vi "PathDrawerMain.vi"() -> ()   [LabVIEW 2017]
uses:
  Dawgma Programming Library/Controls/PurePursuit/PathFileData.ctl
  Dawgma Programming Library/Controls/PurePursuit/RobotNeededPathData.ctl
panel:
  in  "Tab Control":enum32{"Path", "Load/Save"}(tab)
  in  "Deaccel":dbl=50.0 format="%#_13g"
  in  "SlowSpeed":dbl=15.0 format="%#_13g"
  in  "SlowDistanceAtEnd":dbl=12.0 format="%#_13g"
  in  "Speed/Curve":dbl=2.0 format="%#_13g"
  in  "DriveBackwards?":bool
  in  "Lookahead":dbl=13.0
  out "Points (in)":cluster{dbl, dbl}[](array[cluster])=[{14.875179340028694, 248.22955523672883}, {20.874656142200276, 248.30358846723587}, {26.874111844136586, 248.37762105138137}, {32.87350807743945, 248.45164576572313}, {38.87285031681461, 248.52564930010115}, {44.8721376174185, 248.59961966708173}, {50.87132679490307, 248.67354461649725}, {56.87033754344792, 248.74740402354425}, {62.86906734714655, 248.82116341910367}, {68.86738582507886, 248.8947700228471}, {74.8651048928512, 248.9681473786283}, {80.86193607975939, 249.04118420575625}, {86.85743425686633, 249.11371611190245}, {92.85096070503305, 249.18549244057994}, {98.84145913304778, 249.25615421906943}, {104.8276556156584, 249.32512066220386}, {110.80708687815371, 249.39160976611277}, {116.77680979233328, 249.4543515328238}, {122.73186791730424, 249.5115256430506}, {128.6649834222615, 249.56041338385793}, {134.56548779738634, 249.5969246365727}, {140.417375186257, 249.6149706245841}, {146.1966910294908, 249.60548863042237}, {151.86775390690585, 249.55495714900198}, {157.37740484291632, 249.4431992192172}, {162.64635606562646, 249.2401236836006}, {167.55632241578652, 248.9008602167623}, {172.80142342709613, 248.36924030479463}, {178.27099698643164, 247.70868036210402}, {183.89073844553332, 246.9617176111296}, {189.61066276690974, 246.15689887726526}, {195.3970009046773, 245.3134049055755}, {201.22672879119182, 244.44415649854506}, {207.08384341112958, 243.55790546653972}, {212.9567773862825, 242.6606503511154}, {218.83652869344567, 241.75660718632653}, {224.71520193237015, 240.84889249476205}, {230.58472714757215, 239.94002850052652}, {236.43555125878544, 239.03235181687802}, {242.25509137335504, 238.1283916506969}, {248.0256984324822, 237.231278977795}, {253.72180303927817, 236.34525315742894}, {259.30577066584806, 235.47634844945551}, {264.7218219756948, 234.63337048251796}, {269.8869762914892, 233.8293235417345}, {274.67764890352106, 233.08351364924852}, {278.909612625538, 232.42467718794836}]
  in  "Points":cluster{dbl, dbl}[](array[cluster])=[{40.0, 78.0}, {202.0, 76.0}, {324.0, 95.0}]
  in  "Roundedness":dbl(slide)=0.8606565656565657 scale=0.6..0.997
  in  "Length":dbl=38.5
  in  "Width":dbl=33.0
  in  "CenterRotOffset":dbl=15.5
  in  "PointSpacing":dbl=6.0 min=1.0 format="%#_13g"
  in  "Flip Path":bool
  in  "MaxVel":dbl=110.0 format="%#_13g"
  in  "Accel":dbl=50.0 format="%#_13g"
  in  "StartingPosition":enum16{"1", "2", "3", "4", "No Preset"}(ring)
  in  "ExportAllToRobot":bool
  in  "LocalTempPaths":i32(listbox)
  out "standard output":string
  in  "SaveToLocal":bool
  in  "LoadFromLocal":bool
  in  "ExportToRobot":bool
  in  "LoadAllFromRobot":bool
  in  "LocalPaths":i32(listbox)=2
  out "standard error":string="NI Linux Real-Time (run mode)\n\nLog in with your NI-Auth credentials.\n\n"
  in  "LocalFileNames":string[](array[string])=["1A.txt", "1B.txt", "1C.txt", "1D.txt", "2A.txt", "2B.txt", "2C.txt", "2D.txt", "3A.txt", "3B.txt", "3C.txt", "3D.txt", "4A.txt", "4B.txt", "4C.txt", "4D.txt"]
  in  "Stop":bool
  out "Path Drawer":T1(plugin-control)
  # "Includes bumpers"
  # "INSTRUCTIONS"
  # "The red line is the path that the robot recieves. Everything else is to help create that path\n\nUse the multi-line tool to draw a path. Double click to stop drawing.\nHover over a node and press backspace to remove it.\nPress I to insert a new node (at the end of the path only, for now)\n\nUse the contols to input robot width, height, and center of rotation offset,\nHow far apart the points in the \"real world units\" path are,\nWhether the robot travels on the left or right of your green lines, and\nthe roundedness of the path. (Note: point spacing affects roundedness)\n\nYou can manually edit the green node's location in the path with the Points array,\nor drag the nodes on the image\n\nPress Export To File and enter the file name (no extension) to save the path to a file in the\nThisVIsDirectory\\Paths\\ folder\n\nIf you acidentally clear your path press Z quickly to get it back"
  # "Responses of CMDs run"
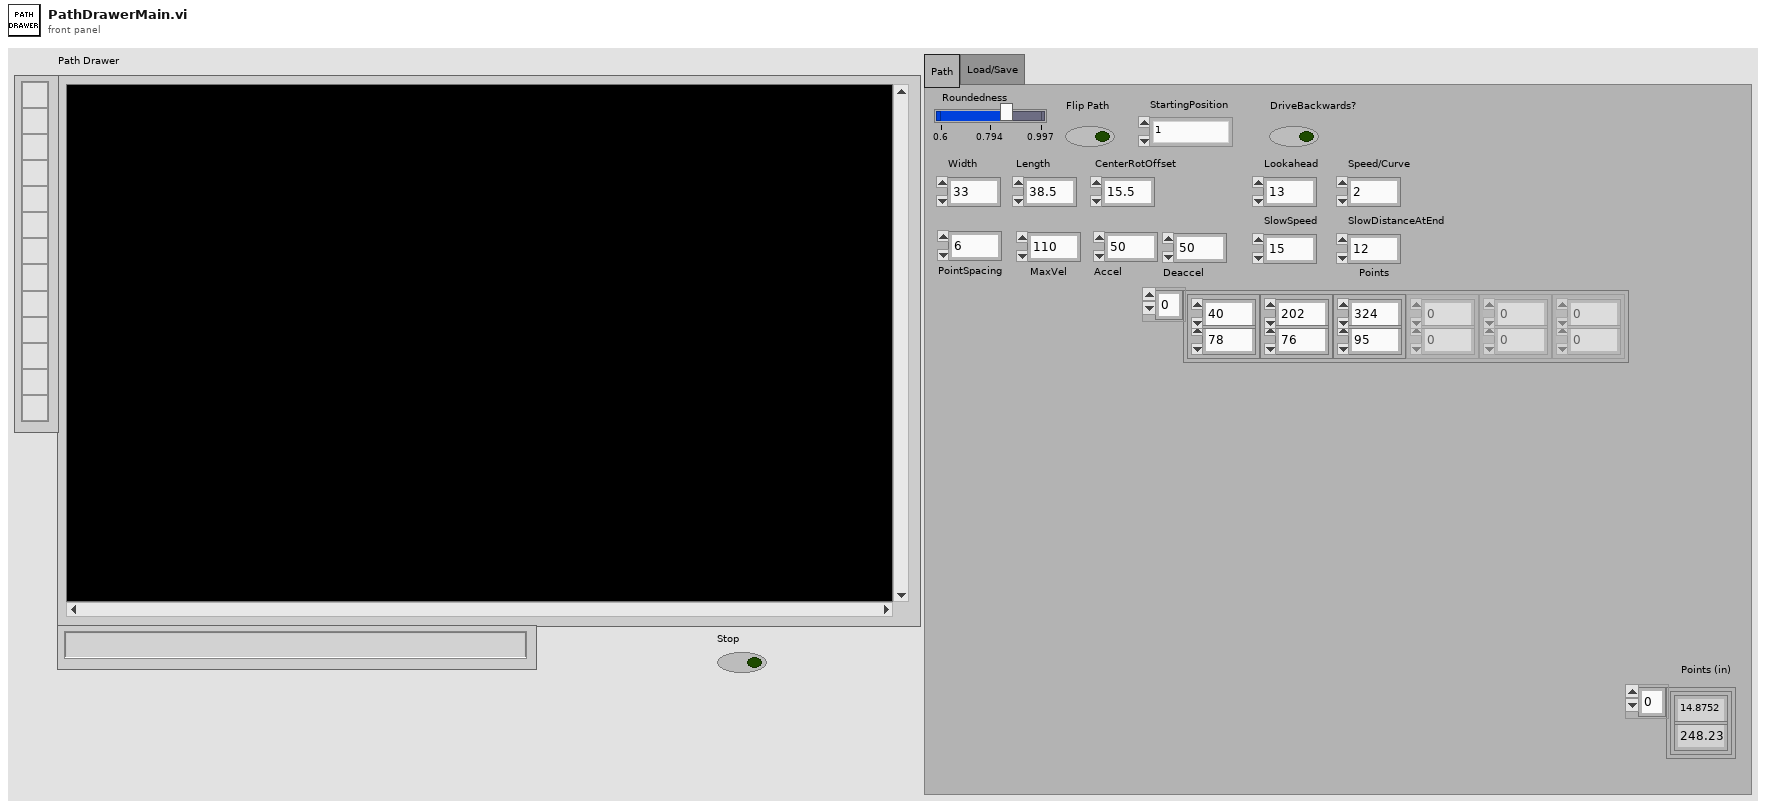
[diagram p1: front panel]
types:
  T1 = typedef "IMAQ Image.ctl" = refnum<image>
  T2 = typedef "Image Type" = u32
  T3 = enum16{"open", "replace", "create", "open or create", "replace or create", "replace or create with confirmation"}
  T4 = cluster{"Global Rectangle":i32[], "Contours":cluster{"Contour Type":u32, "ROI Type":u32, "Points":i32[]}[]}
  T5 = cluster{"Contour Type":u32, "ROI Type":u32, "Points":i32[]}[]
  T6 = cluster{"Contour Type":u32, "ROI Type":u32, "Points":i32[]}
  T7 = typedef "PathFileData.ctl" = cluster{"RobotNeeded":T8, "Meta":cluster{"Path (px)":cluster{i32, i32}[], "RobotWidth":dbl, "RobotLength":dbl, "CenterOfRotYOffset":dbl, "Roundedness":dbl, "StartingPositionPreset":u32, "PathName":string}}
  T8 = typedef "RobotNeededPathData.ctl" = cluster{"Path":cluster{dbl, dbl}[], "MaxVel":dbl, "MaxAccel":dbl, "Backwards?":bool, "PointSpacing":dbl, "LookaheadDist":dbl, "Speed/Curve":dbl, "SlowDistanceAtEnd":dbl, "SlowSpeed":dbl, "MaxDeAccel":dbl}
  T9 = cluster{"Path (px)":cluster{i32, i32}[], "RobotWidth":dbl, "RobotLength":dbl, "CenterOfRotYOffset":dbl, "Roundedness":dbl, "StartingPositionPreset":u32, "PathName":string}
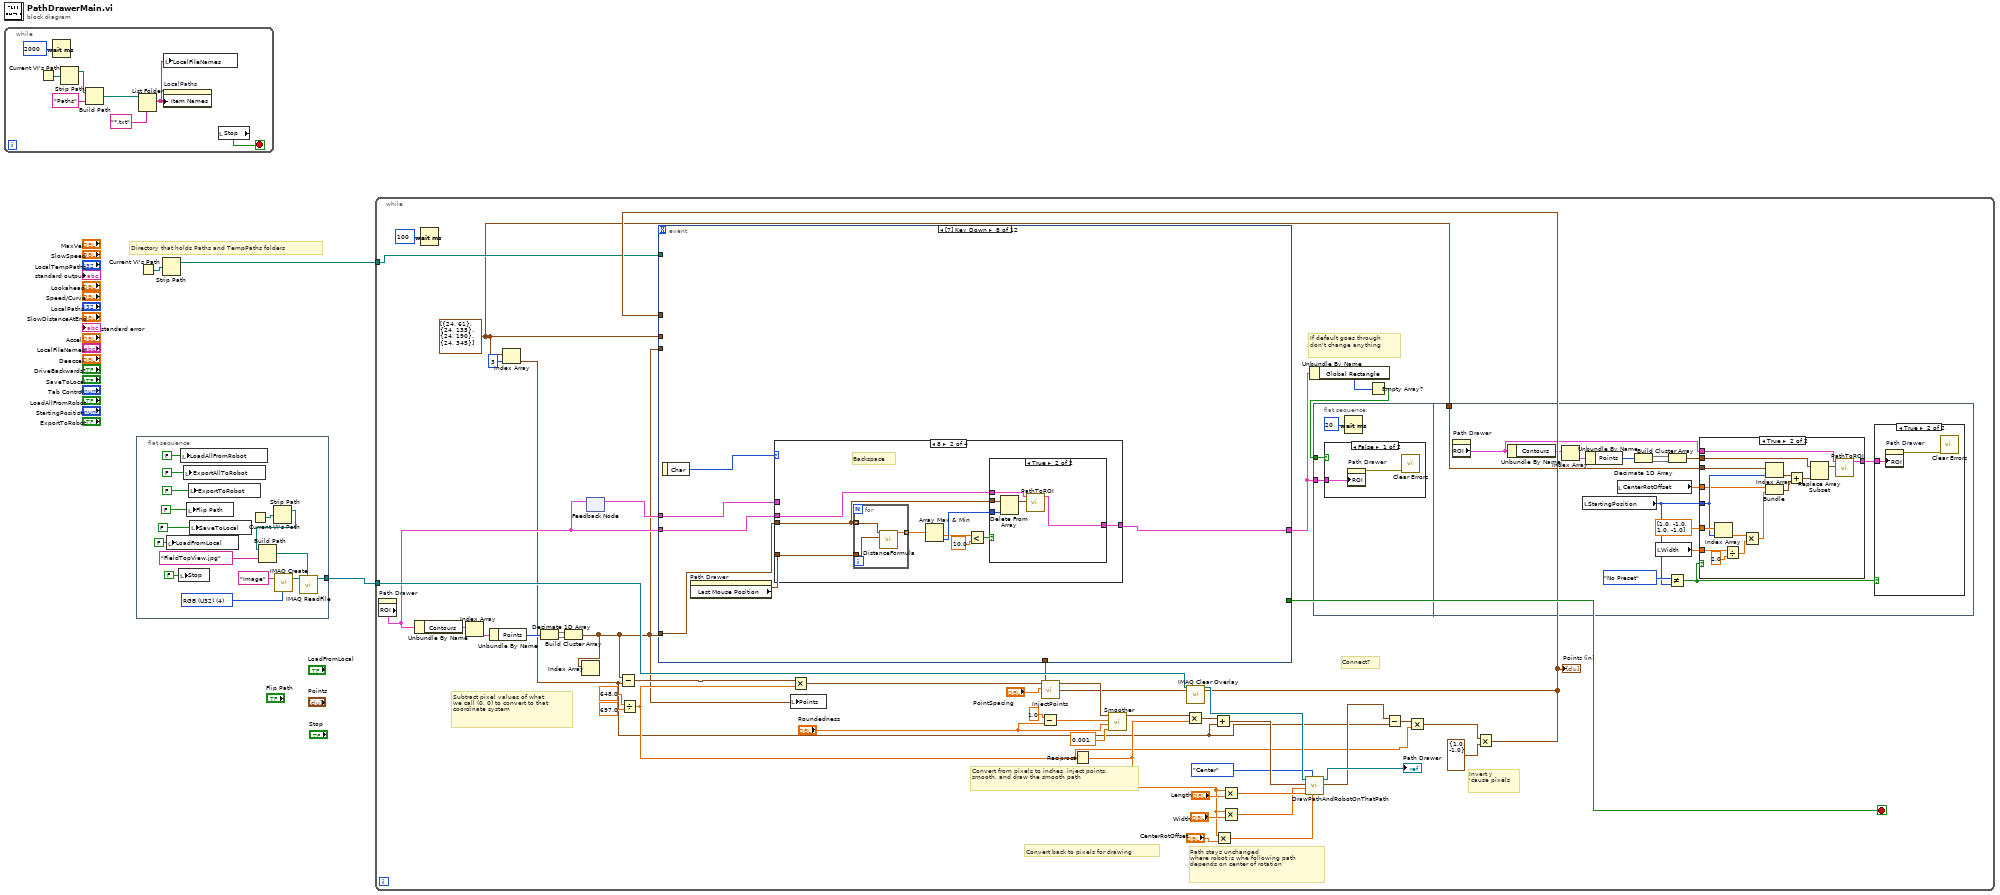
[diagram p0: block diagram]
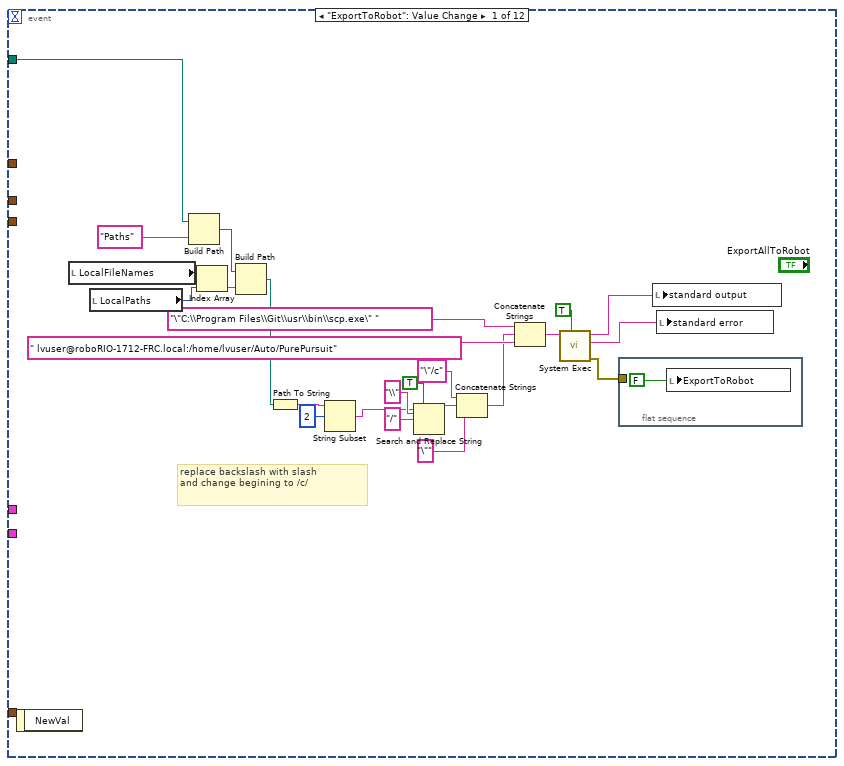
[diagram p5: hidden frame]
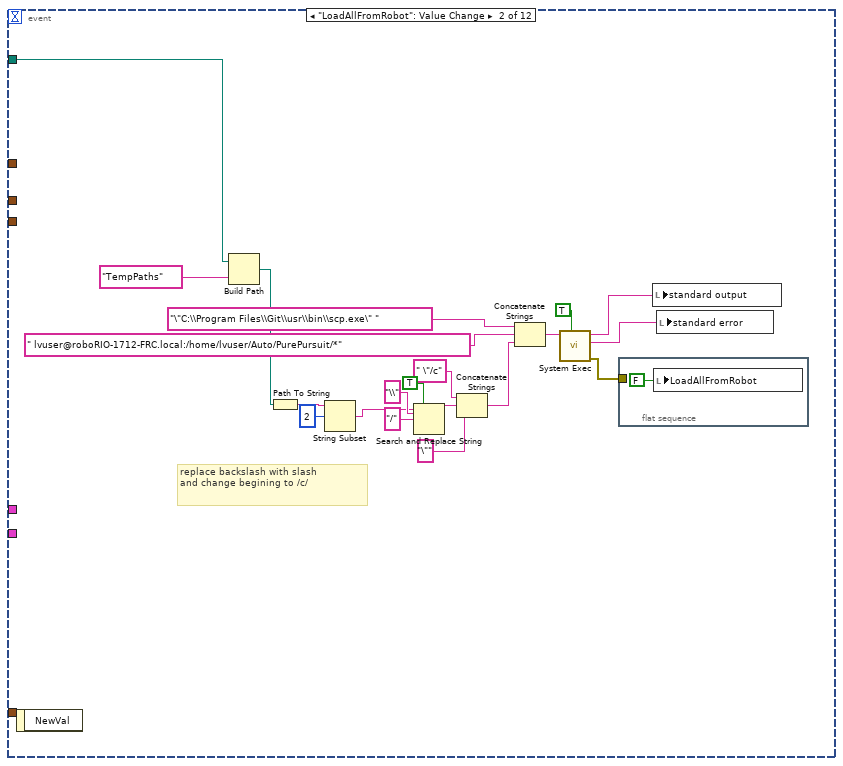
[diagram p6: hidden frame]
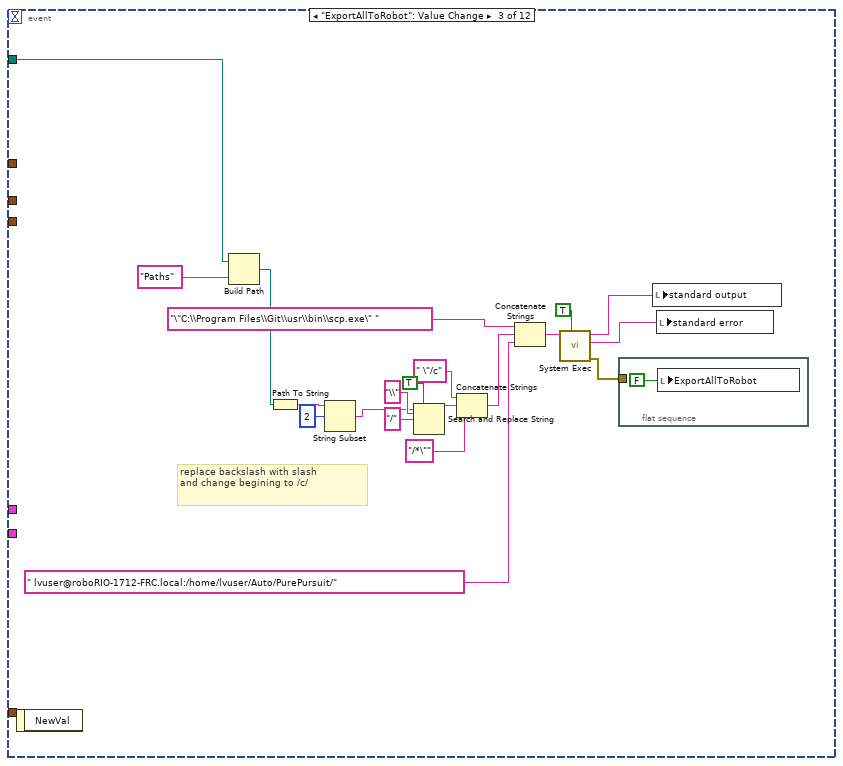
[diagram p7: hidden frame]
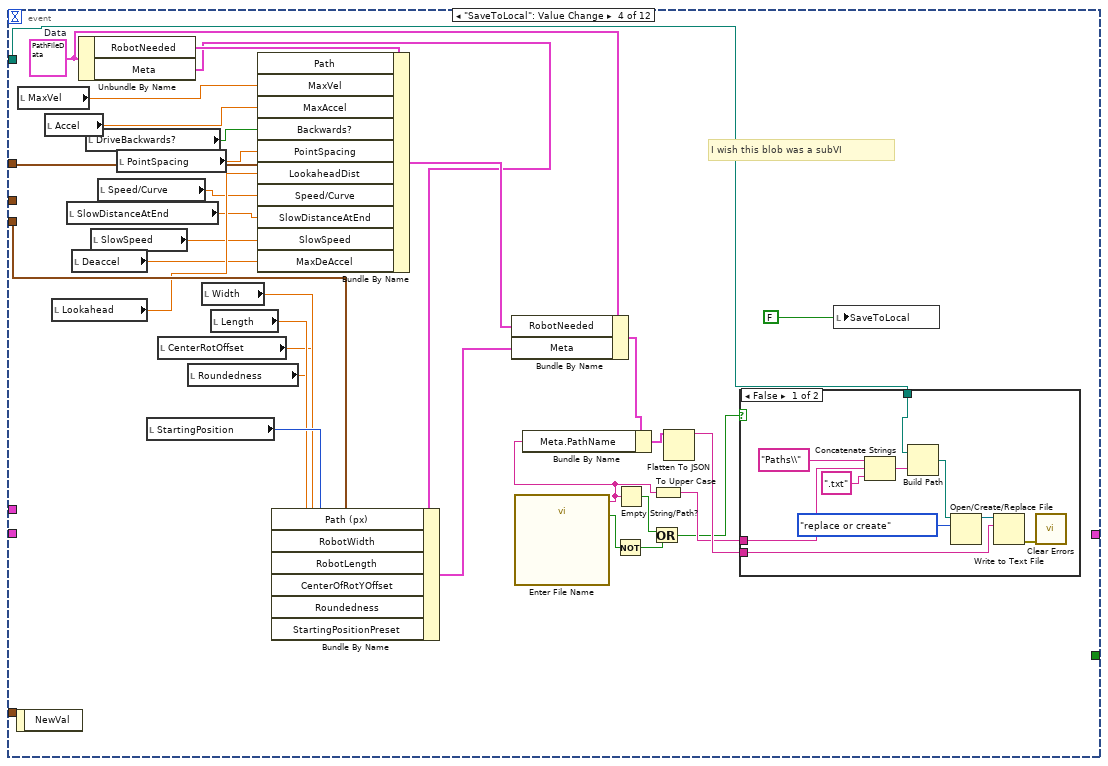
[diagram p8: hidden frame]
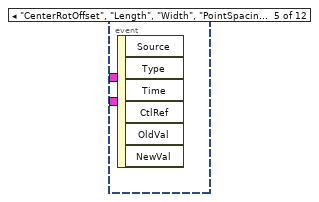
[diagram p10: hidden frame]
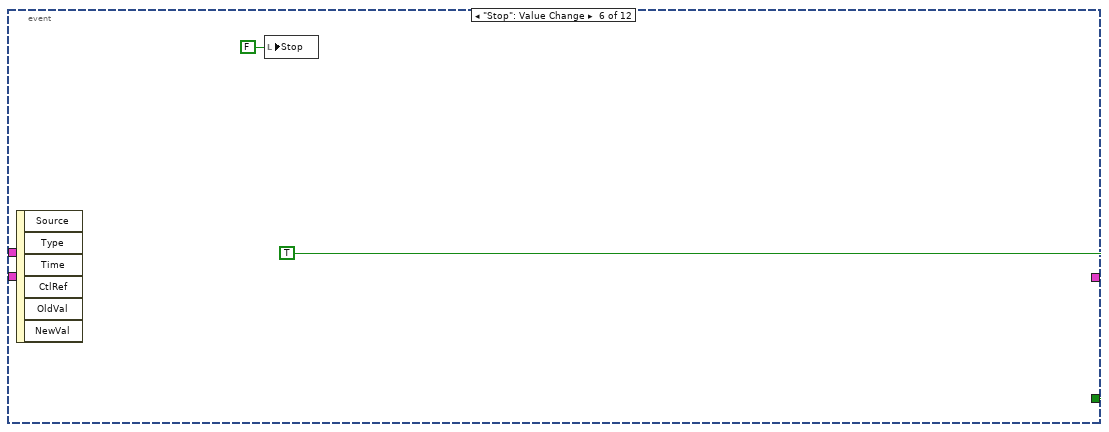
[diagram p11: hidden frame]
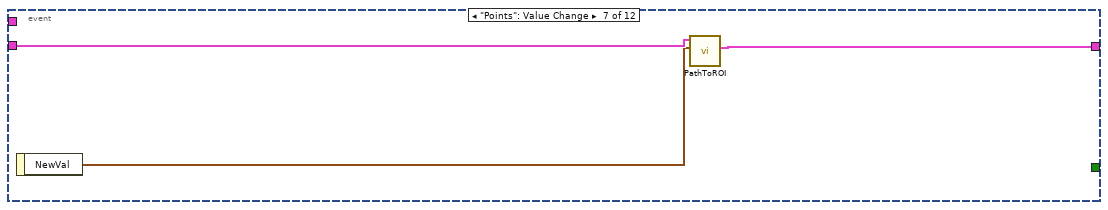
[diagram p12: hidden frame]
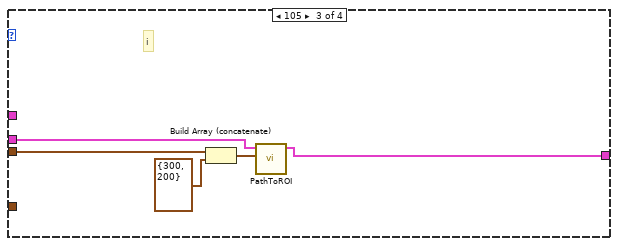
[diagram p15: hidden frame]
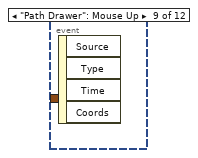
[diagram p17: hidden frame]
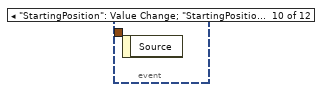
[diagram p18: hidden frame]
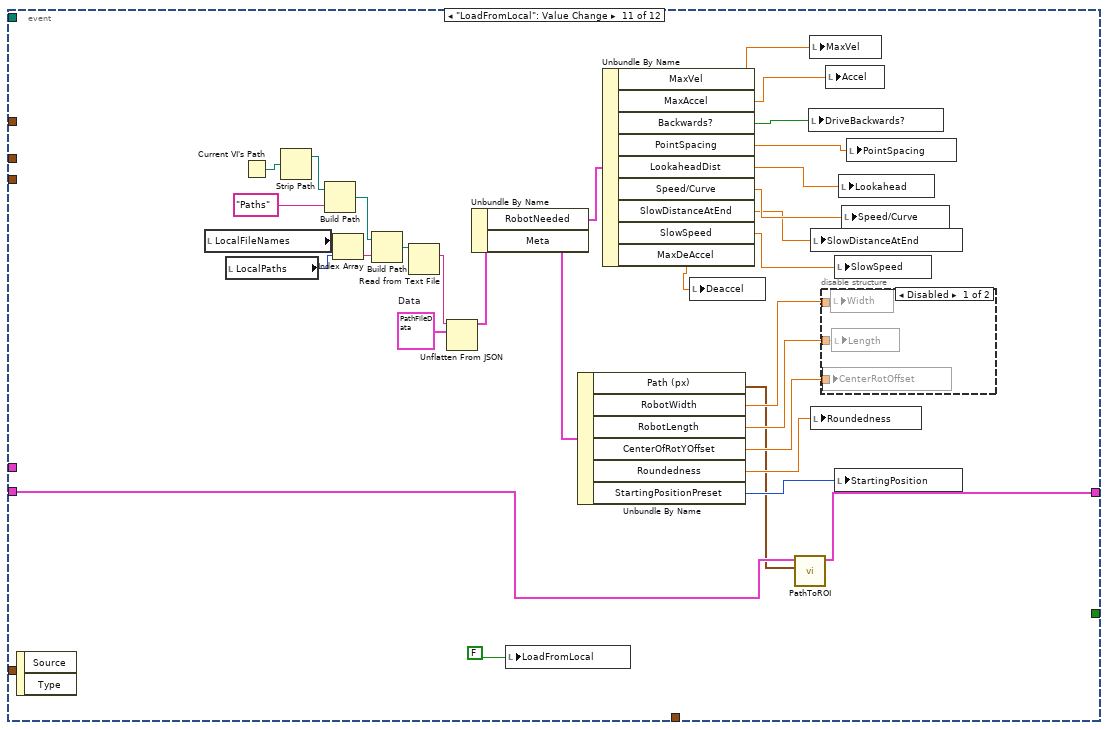
[diagram p19: hidden frame]
diagram:
  # "Directory that holds Paths and TempPaths folders"
  n1 = while {
    stop <- w10 stop-if-true
    n2 = Current VI's Path() -> (path=w5:path)
    n3 = Wait (ms)(milliseconds to wait=u32 2000) -> ()  [unwired: 1 out]
    n4 = Strip Path(path=w5) -> (stripped path=w4:path)  [unwired: 1 out]
    n5 = Build Path(base path=w4, name or relative path="Paths") -> (appended path=w7:path)
    n6 = List Folder(path=w7, pattern="*.txt") -> (filenames=w9:string[])  [unwired: 2 in, 3 out]
    n7 = local write "LocalFileNames"(w9) -> ()
    n8 = property on="LocalPaths" class="LstBox (strict)"("Item Names"=w9) -> ()  [unwired: 2 in, 2 out]
    n9 = local read "Stop"() -> (w10:bool)
  }
  n10 = flat-sequence {
    tunnel: [w21] -> w3
    frame #0 {
      w23 = T2 4 items=["Grayscale (U8)", "Grayscale (I16)", "Grayscale (SGL)", "Complex (CSG)", "RGB (U32)", "HSL (U32)", "RGB (U64)", "Grayscale (U16)"] ("Image Type")
      n11 = local write "LoadFromLocal"(FALSE ("Export To File")) -> ()
      n12 = local write "Stop"(FALSE ("Stop")) -> ()
      n13 = local write "LoadAllFromRobot"(FALSE ("Export To File")) -> ()
      n14 = local write "ExportAllToRobot"(FALSE ("Export To File")) -> ()
      n15 = local write "Flip Path"(FALSE ("Export To File")) -> ()
      n16 = local write "ExportToRobot"(FALSE ("Export To File")) -> ()
      n17 = local write "SaveToLocal"(FALSE ("Export To File")) -> ()
      n18 = Current VI's Path() -> (path=w15:path)
      n19 = Strip Path(path=w15) -> (stripped path=w14:path)  [unwired: 1 out]
      n20 = Build Path(base path=w14, name or relative path="FieldTopView.jpg") -> (appended path=w25:path)
      n21 = call "IMAQ Create"("Image Name"="Image", "Image Type"=w23) -> ("New Image"=w22:T1)  [unwired: 3 in, 1 out]
      n22 = call "IMAQ ReadFile"("File Path"=w25, "Image"=w22) -> ("Image Out"=w21:T1)  [unwired: 5 in, 4 out]
    }
  }
  n23 = Current VI's Path() -> (path=w2:path)
  n24 = Strip Path(path=w2) -> (stripped path=w1:path)  [unwired: 1 out]
  n25 = while {
    tunnel: w3 -> [w67]
    tunnel: w1 -> [w33]
    stop <- w41 stop-if-true
    w27 = cluster{i32, i32}[] [{24, 61}, {24, 135}, {24, 190}, {24, 345}]
    # "Connect?"
    # "Invert y\n'cause pixels"
    # "Path stays unchanged\nwhere robot is whe following path\ndepends on center of rotation"
    # "Convert back to pixels for drawing"
    # "If default goes through\ndon't change anything"
    # "Convert from pixels to inches, inject points,\nsmooth, and draw the smooth path"
    # "Subtract pixel values of what\nwe call (0, 0) to convert to that\ncoordinate system"
    n26 = property on="Path Drawer" class="ImageControl"() -> ("ROI"=w37:T4)  [unwired: 2 in, 2 out]
    n27 = Unbundle By Name(w37) -> ("Contours"=w73:T5)
    n28 = Wait (ms)(milliseconds to wait=u32 100) -> ()  [unwired: 1 out]
    n29 = Index Array(array=w73) -> (element=w68:T6)  [unwired: 1 in]
    n30 = Unbundle By Name(w68) -> ("Points"=w62:i32[])
    n31 = Index Array(array=w27, index=3) -> (element=w31:cluster{i32, i32})
    n32 = Decimate 1D Array(w62) -> (w72:i32[], w71:i32[])
    n33 = Build Cluster Array(w72, w71) -> (w35:cluster{i32, i32}[])
    n34 = Index Array(array=w35) -> ()  [unwired: 1 in, 1 out]
    n35 = feedback-in #1(w37) -> ()
    n36 = feedback #1() -> (w50:T4)  [unwired: 1 in]
    n37 = Subtract(x=w35, y=w31) -> (x-y=w63:cluster{i32, i32}[])
    n38 = Divide(x=648.0, y=697.0) -> (x/y=w38:dbl)
    n39 = local write "Points"(w35) -> ()
    n40 = Multiply(x=w63, y=w38) -> (x*y=w51:cluster{dbl, dbl}[])
    n41 = call "InjectPoints.vi"("Distance"="PointSpacing", "Path"=w51) -> ("Path out"=w65:cluster{dbl, dbl}[])  [unwired: 9 in]
    n42 = Subtract(x=1.0, y="Roundedness") -> (x-y=w60:dbl)
    n43 = Reciprocal(x=w38) -> (1/x=w48:dbl)
    n44 = call "Smoother.vi"("tolerance"=0.001, "B"="Roundedness", "A"=w60, "Path"=w65) -> ("SmoothPath"=w56:cluster{dbl, dbl}[])  [unwired: 7 in]
    n45 = Multiply(x=w56, y=w48) -> (x*y=w64:cluster{dbl, dbl}[])
    n46 = call "IMAQ Clear Overlay"("Image"=w67) -> ("Image Out"=w45:T1)  [unwired: 9 in, 1 out]
    n47 = Add(x=w64, y=w31) -> (x+y=w44:cluster{dbl, dbl}[])
    n48 = Multiply(x=w48, y="CenterRotOffset") -> (x*y=w28:dbl)
    n49 = Multiply(x=w48, y="Length") -> (x*y=w43:dbl)
    n50 = Multiply(x=w48, y="Width") -> (x*y=w29:dbl)
    n51 = call "DrawPathAndRobotOnThatPath.vi"("CenterOfRotYOffset (px)"=w28, "PathMode"=enum16{"Left", "Right", "Center"}."Center", "RobotLength (px)"=w43, "RobotWidth (px)"=w29, "Path (px)"=w44, "Image In"=w45) -> ("NewPath (px)"=w46:cluster{dbl, dbl}[], "Image Out"=→"Path Drawer":T1)  [unwired: 4 in]
    n52 = flat-sequence {
      tunnel: w36 -> [w76]
      tunnel: w30 -> [w75]
      tunnel: w27 -> [w90]
      frame #0 {
        n53 = case shown="False" w75 {
          tunnel: w76 -> [w77 _]
          frame False {
            n54 = property on="Path Drawer" class="ImageControl"("ROI"=w77) -> (error out=w78:errorcluster)  [unwired: 2 in, 1 out]
            n55 = call <vilib>:"Clear Errors.vi"("error in (no error)"=w78) -> ()  [unwired: 5 in, 2 out]
          }
          frame True {
          }
        }
        n56 = Wait (ms)(milliseconds to wait=u32 20) -> ()  [unwired: 1 out]
      }
      frame #1 {
        n57 = property on="Path Drawer" class="ImageControl"() -> ("ROI"=w84:T4)  [unwired: 2 in, 2 out]
        n58 = Unbundle By Name(w84) -> ("Contours"=w85:T5)
        n59 = Index Array(array=w85) -> (element=w88:T6)  [unwired: 1 in]
        n60 = local read "StartingPosition"() -> (w91:enum16{"1", "2", "3", "4", "No Preset"})
        n61 = Unbundle By Name(w88) -> ("Points"=w89:i32[])
        n62 = local read "CenterRotOffset"() -> (w79:dbl)
        n63 = Decimate 1D Array(w89) -> (w86:i32[], w87:i32[])
        n64 = local read "Width"() -> (w80:dbl)
        n65 = Not Equal?(x=enum16{"1", "2", "3", "4", "No Preset"}."No Preset" ("y"), y=w91) -> (x != y?=w81:bool)
        n66 = Build Cluster Array(w86, w87) -> (w83:cluster{i32, i32}[])
        n67 = case shown="True" w81 {
          tunnel: [_ w111] -> w82
          tunnel: w84 -> [_ w110]
          tunnel: w83 -> [_ w108]
          tunnel: w91 -> [_ w98]
          tunnel: w80 -> [_ w102]
          tunnel: w90 -> [_ w101]
          tunnel: dbl[] [1.0, -1.0, 1.0, -1.0] -> [_ w99]
          tunnel: w79 -> [_ w96]
          frame False {
          }
          frame True {
            n68 = Index Array(array=w99, index=w98) -> (element=w97:dbl)
            n69 = Divide(x=w102, y=2.0) -> (x/y=w105:dbl)
            n70 = Multiply(x=w97, y=w105) -> (x*y=w104:dbl)
            n71 = Index Array(array=w101, index=w98) -> (element=w100:cluster{i32, i32})
            n72 = Bundle("CenterRotOffset"=w96, w104) -> (w103:cluster{"CenterRotOffset":dbl, dbl})  [unwired: 1 in]
            n73 = Add(x=w100, y=w103) -> (x+y=w107:cluster{dbl, dbl})
            n74 = Replace Array Subset(array=w108, new element=w107) -> (w109:cluster{i32, i32}[])  [unwired: 1 in]
            n75 = call "PathToROI.vi"("Path In"=w109, "ROI In"=w110) -> ("ROI Out"=w111:T4)  [unwired: 9 in]
          }
        }
        n76 = case shown="True" w81 {
          tunnel: w82 -> [_ w94]
          frame False {
          }
          frame True {
            n77 = property on="Path Drawer" class="ImageControl"("ROI"=w94) -> (error out=w95:errorcluster)  [unwired: 2 in, 1 out]
            n78 = call <vilib>:"Clear Errors.vi"("error in (no error)"=w95) -> ()  [unwired: 5 in, 2 out]
          }
        }
      }
    }
    n79 = Subtract(x=w46, y=w31) -> (x-y=w52:cluster{dbl, dbl}[])
    n80 = Multiply(x=w52, y=w38) -> (x*y=w40:cluster{dbl, dbl}[])
    n81 = Multiply(x=w40, y=cluster{dbl, dbl} {1.0, -1.0}) -> (x*y=w34:cluster{dbl, dbl}[])
    "Points (in)" <- w34
    n82 = event shown="[7] Key Down" {
      selector: _ -> [_ _ _ _ _ _ _ _ _ _ _ _]
      dyn-events: _ -> [_ _ _ _ _ _ _ _ _ _ _ _]
      timeout: _ -> [_ _ _ _ _ _ _ _ _ _ _ _]
      tunnel: w37 -> [_ _ _ _ _ _ w225 w231 _ _ w272 w302]
      tunnel: [_ _ _ _ _ _ w224 w228 _ _ w286 w301] -> w36
      tunnel: w34 -> [_ _ _ _ _ _ _ _ _ _ _ _]
      tunnel: w50 -> [_ _ _ _ _ _ _ w227 _ _ _ _]
      tunnel: w35 -> [_ _ _ _ _ _ _ w226 _ _ _ w296]
      tunnel: [_ _ _ _ _ TRUE ("Stop") _ _ _ _ _ _] -> w41
      tunnel: w35 -> [_ _ _ w194 _ _ _ _ _ _ _ _]
      tunnel: w34 -> [_ _ _ w193 _ _ _ _ _ _ _ _]
      tunnel: w33 -> [w112 w137 w158 w186 _ _ _ _ _ _ _ _]
      tunnel: w27 -> [_ _ _ _ _ _ _ _ _ _ _ _]
      event "ExportToRobot": Value Change {
        # "replace backslash with slash\nand change begining to /c/"
        n83 = event-data() -> ()  [unwired: 1 in, 1 out]
        n84 = local read "LocalFileNames"() -> (w119:string[])
        n85 = local read "LocalPaths"() -> (w120:i32)
        n86 = Build Path(base path=w112, name or relative path="Paths") -> (appended path=w122:path)
        n87 = Index Array(array=w119, index=w120) -> (element=w121:string)
        n88 = Build Path(base path=w122, name or relative path=w121) -> (appended path=w117:path)
        n89 = Path To String(path=w117) -> (string=w128:string)
        n90 = String Subset(string=w128, offset (0)=2) -> (substring=w126:string)  [unwired: 1 in]
        n91 = Search and Replace String(replace all?=TRUE ("replace all? (F)"), input string=w126, search string="\\", replace string="/" ("replace string (\"\")")) -> (result string=w125:string)  [unwired: 4 in, 3 out]
        n92 = Concatenate Strings("\"/c" ("string"), w125, "\"" ("string")) -> (w123:string)
        n93 = Concatenate Strings("\"C:\\Program Files\\Git\\usr\\bin\\scp.exe\" " ("command line"), w123, " lvuser@roboRIO-1712-FRC.local:/home/lvuser/Auto/PurePursuit" ("string")) -> (w132:string)
        n94 = call <vilib>:"System Exec.vi"("wait until completion? (T)"=TRUE, "command line"=w132) -> ("error out"=w115:errorcluster, "standard error"=w113:string, "standard output"=w114:string)  [unwired: 6 in, 1 out]
        n95 = flat-sequence {
          tunnel: w115 -> [_]
          frame #0 {
            n96 = local write "ExportToRobot"(FALSE ("Export To File")) -> ()
          }
        }
        n97 = local write "standard output"(w114) -> ()
        n98 = local write "standard error"(w113) -> ()
      }
      event "LoadAllFromRobot": Value Change {
        # "replace backslash with slash\nand change begining to /c/"
        n99 = event-data() -> ()  [unwired: 1 in, 1 out]
        n100 = Build Path(base path=w137, name or relative path="TempPaths") -> (appended path=w140:path)
        n101 = Path To String(path=w140) -> (string=w150:string)
        n102 = String Subset(string=w150, offset (0)=2) -> (substring=w148:string)  [unwired: 1 in]
        n103 = Search and Replace String(replace all?=TRUE ("replace all? (F)"), input string=w148, search string="\\", replace string="/" ("replace string (\"\")")) -> (result string=w147:string)  [unwired: 4 in, 3 out]
        n104 = Concatenate Strings(" \"/c" ("string"), w147, "\"" ("string")) -> (w138:string)
        n105 = Concatenate Strings("\"C:\\Program Files\\Git\\usr\\bin\\scp.exe\" " ("command line"), " lvuser@roboRIO-1712-FRC.local:/home/lvuser/Auto/PurePursuit/*" ("string"), w138) -> (w154:string)
        n106 = call <vilib>:"System Exec.vi"("wait until completion? (T)"=TRUE, "command line"=w154) -> ("error out"=w143:errorcluster, "standard error"=w141:string, "standard output"=w142:string)  [unwired: 6 in, 1 out]
        n107 = flat-sequence {
          tunnel: w143 -> [_]
          frame #0 {
            n108 = local write "LoadAllFromRobot"(FALSE ("Export To File")) -> ()
          }
        }
        n109 = local write "standard output"(w142) -> ()
        n110 = local write "standard error"(w141) -> ()
      }
      event "ExportAllToRobot": Value Change {
        # "replace backslash with slash\nand change begining to /c/"
        n111 = event-data() -> ()  [unwired: 1 in, 1 out]
        n112 = Build Path(base path=w158, name or relative path="Paths") -> (appended path=w161:path)
        n113 = Path To String(path=w161) -> (string=w171:string)
        n114 = String Subset(string=w171, offset (0)=2) -> (substring=w169:string)  [unwired: 1 in]
        n115 = Search and Replace String(replace all?=TRUE ("replace all? (F)"), input string=w169, search string="\\", replace string="/" ("replace string (\"\")")) -> (result string=w168:string)  [unwired: 4 in, 3 out]
        n116 = Concatenate Strings(" \"/c" ("string"), w168, "/*\"" ("string")) -> (w160:string)
        n117 = Concatenate Strings("\"C:\\Program Files\\Git\\usr\\bin\\scp.exe\" " ("command line"), w160, " lvuser@roboRIO-1712-FRC.local:/home/lvuser/Auto/PurePursuit/" ("string")) -> (w175:string)
        n118 = call <vilib>:"System Exec.vi"("wait until completion? (T)"=TRUE, "command line"=w175) -> ("error out"=w164:errorcluster, "standard error"=w162:string, "standard output"=w163:string)  [unwired: 6 in, 1 out]
        n119 = flat-sequence {
          tunnel: w164 -> [_]
          frame #0 {
            n120 = local write "ExportAllToRobot"(FALSE ("Export To File")) -> ()
          }
        }
        n121 = local write "standard output"(w163) -> ()
        n122 = local write "standard error"(w162) -> ()
      }
      event "SaveToLocal": Value Change {
        w192 = T7 {"RobotNeeded"={"Path"=[], "MaxVel"=0.0, "MaxAccel"=0.0, "Backwards?"=FALSE, "PointSpacing"=0.0, "LookaheadDist"=0.0, "Speed/Curve"=1.8, "SlowDistanceAtEnd"=12.0, "SlowSpeed"=15.0, "MaxDeAccel"=0.0}, "Meta"={"Path (px)"=[], "RobotWidth"=0.0, "RobotLength"=0.0, "CenterOfRotYOffset"=0.0, "Roundedness"=0.0, "StartingPositionPreset"=2, "PathName"=""}}  # Data
        # "I wish this blob was a subVI"
        n123 = event-data() -> ()  [unwired: 1 in, 1 out]
        n124 = local read "MaxVel"() -> (w185:dbl)
        n125 = local read "Accel"() -> (w184:dbl)
        n126 = local read "Lookahead"() -> (w188:dbl)
        n127 = local read "SlowDistanceAtEnd"() -> (w181:dbl)
        n128 = local read "Deaccel"() -> (w179:dbl)
        n129 = Unbundle By Name(w192) -> ("RobotNeeded"=w201:T8, "Meta"=w200:T9)
        n130 = local read "DriveBackwards?"() -> (w187:bool)
        n131 = local read "SlowSpeed"() -> (w180:dbl)
        n132 = local read "Speed/Curve"() -> (w182:dbl)
        n133 = local read "PointSpacing"() -> (w204:dbl)
        n134 = local read "StartingPosition"() -> (w203:enum16{"1", "2", "3", "4", "No Preset"})
        n135 = local read "CenterRotOffset"() -> (w196:dbl)
        n136 = local read "Roundedness"() -> (w195:dbl)
        n137 = local read "Width"() -> (w198:dbl)
        n138 = local read "Length"() -> (w197:dbl)
        n139 = Bundle By Name(cluster=w201, "Path"=w193, "MaxVel"=w185, "MaxAccel"=w184, "Backwards?"=w187, "PointSpacing"=w204, "LookaheadDist"=w188, "Speed/Curve"=w182, "SlowDistanceAtEnd"=w181, "SlowSpeed"=w180, "MaxDeAccel"=w179) -> (w202:T8)
        n140 = Bundle By Name(cluster=w200, "Path (px)"=w194, "RobotWidth"=w198, "RobotLength"=w197, "CenterOfRotYOffset"=w196, "Roundedness"=w195, "StartingPositionPreset"=w203) -> (w199:T9)
        n141 = Bundle By Name(cluster=w192, "RobotNeeded"=w202, "Meta"=w199) -> (w191:T7)
        n142 = call "Enter File Name"() -> ("File Name"=w190:string, "Enter"=w206:bool)  [unwired: 17 in, 1 out]
        n143 = Bundle By Name(cluster=w191, "Meta.PathName"=w190) -> (w208:T7)
        n144 = Not(x=w206) -> (.not. x?=w205:bool)
        n145 = Empty String/Path?(string/path=w190) -> (empty?=w207:bool)
        n146 = Or(x=w207, y=w205) -> (x .or. y?=w183:bool)
        n147 = To Upper Case(1:w190) -> (0:w189:string)
        n148 = Flatten To JSON(anything=w208) -> (JSON string=w209:string)  [unwired: 2 in, 1 out]
        n149 = case shown="False" w183 {
          tunnel: w189 -> [w216 _]
          tunnel: w209 -> [w215 _]
          tunnel: w186 -> [w211 _]
          frame False {
            n150 = Concatenate Strings("Paths\\" ("name or relative path"), w216, ".txt" ("string")) -> (w220:string)
            n151 = Build Path(base path=w211, name or relative path=w220) -> (appended path=w214:path)
            n152 = Open/Create/Replace File(file path (use dialog)=w214, operation (0:open)=T3."replace or create") -> (refnum out=w213:refnum<file>)  [unwired: 4 in, 2 out]
            n153 = Write to Text File(file (use dialog)=w213, text=w215) -> (error out=w218:errorcluster)  [unwired: 2 in, 2 out]
            n154 = call <vilib>:"Clear Errors.vi"("error in (no error)"=w218) -> ()  [unwired: 5 in, 2 out]
          }
          frame True {
          }
        }
        n155 = local write "SaveToLocal"(FALSE ("Export To File")) -> ()
      }
      event "CenterRotOffset", "Length", "Width", "PointSpacing", "Roundedness": Value Change {
        n156 = event-data() -> ()  [unwired: 1 in, 6 out]
      }
      event "Stop": Value Change {
        n157 = event-data() -> ()  [unwired: 1 in, 6 out]
        n158 = local write "Stop"(FALSE ("Stop")) -> ()
      }
      event "Points": Value Change {
        n159 = event-data() -> ("NewVal"=w223:cluster{dbl, dbl}[])  [unwired: 1 in]
        n160 = call "PathToROI.vi"("Path In"=w223, "ROI In"=w225) -> ("ROI Out"=w224:T4)  [unwired: 9 in]
      }
      event Key Down {
        n161 = event-data() -> ("Char"=w230:i16)  [unwired: 1 in]
        n162 = property on="Path Drawer" class="ImageControl"() -> ("Last Mouse Position"=w229:cluster{"X":i32, "Y":i32})  [unwired: 2 in, 2 out]
        n163 = case shown="8" w230 {
          tunnel: w231 -> [w232 w241 w253 _]
          tunnel: w226 -> [_ w240 w255 _]
          tunnel: w229 -> [_ w234 _ _]
          tunnel: [w232 w233 w251 w256] -> w228
          tunnel: w227 -> [_ _ _ w256]
          frame 0, Default {
          }
          frame 8 {
            # "Backspace"
            n164 = for {
              tunnel: w240 -> [w250] mode=indexing
              tunnel: [w249] -> w239 mode=indexing
              tunnel: w234 -> [w248]
              n165 = call "DistanceFormula.vi"("Point 2"=w248, "Point 1"=w250) -> ("Distance"=w249:dbl)  [unwired: 9 in]
            }
            n166 = Array Max & Min(array=w239) -> (min value=w237:dbl, min index (indices)=w238:i32)  [unwired: 2 out]
            n167 = Less?(x=w237, y=10.0) -> (x < y?=w235:bool)
            n168 = case shown="True" w235 {
              tunnel: w238 -> [_ w247]
              tunnel: w240 -> [_ w246]
              tunnel: w241 -> [w242 w244]
              tunnel: [w242 w243] -> w233
              frame False {
              }
              frame True {
                n169 = Delete From Array(array=w246, index=w247) -> (array with subset deleted=w245:cluster{i32, i32}[])  [unwired: 1 in, 1 out]
                n170 = call "PathToROI.vi"("Path In"=w245, "ROI In"=w244) -> ("ROI Out"=w243:T4)  [unwired: 9 in]
              }
            }
          }
          frame 105 {
            # "i"
            n171 = Build Array (concatenate)(w255, cluster{i32, i32} {300, 200}) -> (w254:cluster{i32, i32}[])
            n172 = call "PathToROI.vi"("Path In"=w254, "ROI In"=w253) -> ("ROI Out"=w251:T4)  [unwired: 9 in]
          }
          frame 122 {
            # "Restore last ROI"
            # "Z"
          }
        }
      }
      event "Path Drawer": Mouse Up {
        n173 = event-data() -> ()  [unwired: 1 in, 4 out]
      }
      event "StartingPosition": Value Change; "StartingPosition": Mouse Down {
        n174 = event-data() -> ()  [unwired: 1 in, 1 out]
      }
      event "LoadFromLocal": Value Change {
        w283 = T7 {"RobotNeeded"={"Path"=[], "MaxVel"=0.0, "MaxAccel"=0.0, "Backwards?"=FALSE, "PointSpacing"=0.0, "LookaheadDist"=0.0, "Speed/Curve"=1.8, "SlowDistanceAtEnd"=12.0, "SlowSpeed"=15.0, "MaxDeAccel"=0.0}, "Meta"={"Path (px)"=[], "RobotWidth"=0.0, "RobotLength"=0.0, "CenterOfRotYOffset"=0.0, "Roundedness"=0.0, "StartingPositionPreset"=2, "PathName"=""}}  # Data
        n175 = event-data() -> ()  [unwired: 1 in, 2 out]
        n176 = local read "LocalFileNames"() -> (w267:string[])
        n177 = local read "LocalPaths"() -> (w268:i32)
        n178 = Current VI's Path() -> (path=w270:path)
        n179 = Strip Path(path=w270) -> (stripped path=w269:path)  [unwired: 1 out]
        n180 = Build Path(base path=w269, name or relative path="Paths") -> (appended path=w275:path)
        n181 = Index Array(array=w267, index=w268) -> (element=w274:string)
        n182 = Build Path(base path=w275, name or relative path=w274) -> (appended path=w273:path)
        n183 = Read from Text File(file (use dialog)=w273) -> (text=w285:string)  [unwired: 3 in, 3 out]
        n184 = Unflatten From JSON(JSON string=w285, type and defaults=w283) -> (value=w282:T7)  [unwired: 5 in, 1 out]
        n185 = Unbundle By Name(w282) -> ("RobotNeeded"=w266:T8, "Meta"=w281:T9)
        n186 = local write "LoadFromLocal"(FALSE ("Export To File")) -> ()
        n187 = Unbundle By Name(w281) -> ("Path (px)"=w271:cluster{i32, i32}[], "RobotWidth"=w276:dbl, "RobotLength"=w277:dbl, "CenterOfRotYOffset"=w280:dbl, "Roundedness"=w279:dbl, "StartingPositionPreset"=w278:u32)
        n188 = Unbundle By Name(w266) -> ("MaxVel"=w265:dbl, "MaxAccel"=w264:dbl, "Backwards?"=w263:bool, "PointSpacing"=w262:dbl, "LookaheadDist"=w261:dbl, "Speed/Curve"=w260:dbl, "SlowDistanceAtEnd"=w259:dbl, "SlowSpeed"=w258:dbl, "MaxDeAccel"=w257:dbl)
        n189 = local write "Deaccel"(w257) -> ()
        n190 = call "PathToROI.vi"("Path In"=w271, "ROI In"=w272) -> ("ROI Out"=w286:T4)  [unwired: 9 in]
        n191 = local write "DriveBackwards?"(w263) -> ()
        n192 = local write "MaxVel"(w265) -> ()
        n193 = local write "SlowDistanceAtEnd"(w259) -> ()
        n194 = local write "Roundedness"(w279) -> ()
        n195 = disable-structure shown="Disabled" {
          disable-tunnel: w280 -> [w290 _]
          disable-tunnel: w277 -> [w289 _]
          disable-tunnel: w276 -> [w288 _]
          frame Disabled {
            n196 = local write "CenterRotOffset"(w290) -> ()
            n197 = local write "Width"(w288) -> ()
            n198 = local write "Length"(w289) -> ()
          }
          frame Enabled {
          }
        }
        n199 = local write "Accel"(w264) -> ()
        n200 = local write "SlowSpeed"(w258) -> ()
        n201 = local write "StartingPosition"(w278) -> ()
        n202 = local write "Lookahead"(w261) -> ()
        n203 = local write "Speed/Curve"(w260) -> ()
        n204 = local write "PointSpacing"(w262) -> ()
      }
      event "Flip Path": Value Change {
        w298 = cluster{i32, i32} {0, 203}
        # "Center of field"
        n205 = event-data() -> ()  [unwired: 1 in, 2 out]
        n206 = local read "StartingPosition"() -> (w292:enum16{"1", "2", "3", "4", "No Preset"})
        n207 = local write "Flip Path"(FALSE ("Export To File")) -> ()
        n208 = Not Equal?(x=enum16{"1", "2", "3", "4", "No Preset"}."No Preset", y=w292) -> (x != y?=w293:bool)
        n209 = Subtract(x=w296, y=w298) -> (x-y=w297:cluster{i32, i32}[])
        n210 = case shown="True" w293 {
          tunnel: w292 -> [w304 w307]
          tunnel: [w304 w305] -> w291
          frame False {
          }
          frame True {
            n211 = Subtract(x=3, y=w307) -> (x-y=w305:i32)
          }
        }
        n212 = Multiply(x=w297, y=cluster{i32, i32} {1, -1}) -> (x*y=w299:cluster{i32, i32}[])
        n213 = Add(x=w299, y=w298) -> (x+y=w295:cluster{i32, i32}[])
        n214 = call "PathToROI.vi"("Path In"=w295, "ROI In"=w302) -> ("ROI Out"=w301:T4)  [unwired: 9 in]
        n215 = local write "StartingPosition"(w291) -> ()
      }
    }
    n216 = Unbundle By Name(w36) -> ("Global Rectangle"=w57:i32[])
    n217 = Empty Array?(array=w57) -> (empty?=w30:bool)
  }
